vi "Circle_Geometry_Solution.vi"(4 "Radius":dbl) -> (0 "Area":dbl, 1 "Circumference":dbl, 2 "Diameter":dbl)   [LabVIEW 2013]
panel:
  # "Circle Geometery\n\nCreate a VI that takes the radius of a circle as an input and\n computes the Diameter, Circumference and Area the circle."
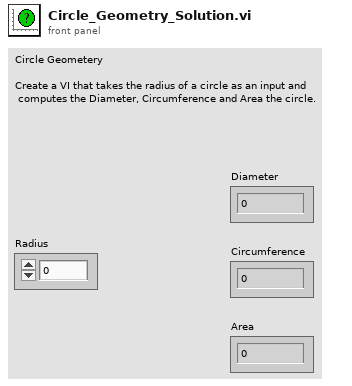
[diagram p1: front panel]
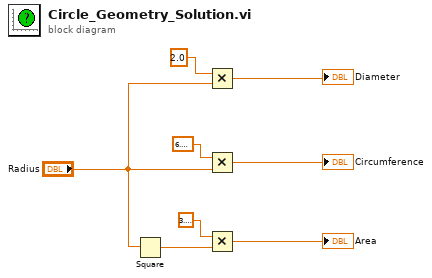
[diagram p0: block diagram]
diagram:
  n1 = Square(x="Radius") -> (x^2=w1:dbl)
  n2 = Multiply(x=2.0, y="Radius") -> (x*y=→"Diameter":dbl)
  n3 = Multiply(x=6.283185307179586, y="Radius") -> (x*y=→"Circumference":dbl)
  n4 = Multiply(x=3.141592653589793, y=w1) -> (x*y=→"Area":dbl)
